vi "Add Shared Approval File and Folder.vi"   [LabVIEW 2020, in "Approval Tests.lvlib"]
doc: "Drops everything needed to put recieved files into a separate folder and still share approved files."
uses:
  Approval Tests.lvlib
  Options/Options.lvclass
  Namer With Shared Approved File/Namer With Shared Approved File.lvclass
  C:/Users/SAS/Desktop/ApprovalTests.LabVIEW/Source/Approval Tests/Namer Decorator/Namer Decorator.lvclass
  Namer with Folder/Namer with Folder.lvclass
  C:/Users/SAS/Desktop/ApprovalTests.LabVIEW/Source/Approval Tests/Namer/Namer.lvclass
  Namer With Shared Approved File/Namer With Shared Approved File.lvclass/Namer With Shared Approved File.ctl
  Namer Decorator/Namer Decorator.lvclass/Namer Decorator.ctl
  Namer With Shared Approved File/Write Shared Approved File Path.vi
  Namer Decorator/Write Decorate.vi
  Options/Write Namer.vi
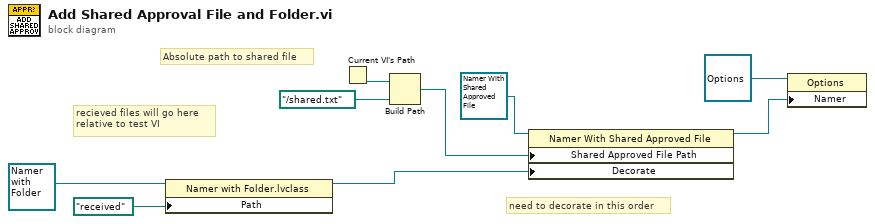
[diagram p0: block diagram]
diagram:
  # "need to decorate in this order"
  # "recieved files will go here\nrelative to test VI"
  # "Absolute path to shared file"
  n1 = property class="Namer with Folder.lvclass"(reference=refnum<class "Namer with Folder.lvclass"> refnum ("Approval Tests:Namer with Folder.lvclass"), "Path"=path "received") -> (reference out=w1:refnum<class "Namer with Folder.lvclass">)  [unwired: 1 in, 1 out]
  n2 = Current VI's Path() -> (path=w6:path)
  n3 = Build Path(base path=w6, name or relative path=path "../shared.txt" ("Path")) -> (appended path=w4:path)
  n4 = property class="Namer With Shared Approved File"(reference=refnum<class "Namer With Shared Approved File.lvclass"> refnum ("Approval Tests.lvlib:Regex Scrubber"), "Shared Approved File Path"=w4, "Decorate"=w1) -> (reference out=w7:refnum<class "Namer With Shared Approved File.lvclass">)  [unwired: 1 in, 1 out]
  n5 = property class="Options"(reference=refnum<class "Options.lvclass"> refnum ("Approval Tests.lvlib:Options"), "Namer"=w7) -> ()  [unwired: 1 in, 2 out]
